vi "Get_Motor_Coordinates.vi"(6 "Microsteps (MS=64)":dbl=64.0, 9 "Output Unit":T1=enum."Micron", 11 "string":string) -> (0 "Motor 4 Coordinate (deg)":dbl, 1 "Motor 3 Coordinate":dbl, 2 "Motor 2 Coordinate":dbl, 3 "Motor 1 Coordinate":dbl)   [LabVIEW 2018]
uses:
  ConversionAndInformation/Unit_Control.ctl
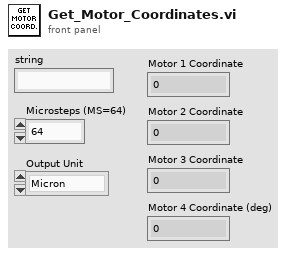
[diagram p1: front panel]
types:
  T1 = typedef "Unit_Control.ctl" = enum16{"Angle (Degrees)", "Rad", "Angle [TMC]", "Microsteps [TMC]", "Inches", "Nanometer", "Meter", "Centimeter", "Millimeter", "Micron"}
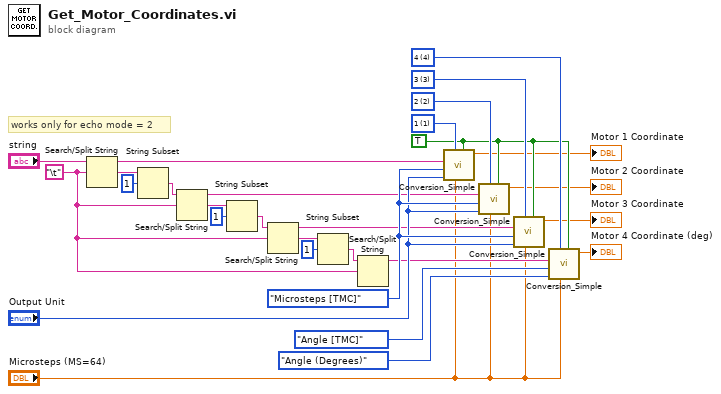
[diagram p0: block diagram]
diagram:
  w7 = u16 4 items=["none", "1", "2", "3", "4", "all"] ("Motor")
  w8 = u16 3 items=["none", "1", "2", "3", "4", "all"] ("Motor")
  w9 = u16 2 items=["none", "1", "2", "3", "4", "all"] ("Motor")
  w10 = u16 1 items=["none", "1", "2", "3", "4", "all"] ("Motor")
  w6 = TRUE ("Input = DBL/String (DBL[false])")
  w18 = Unit_Control."Microsteps [TMC]" ("Output Unit")
  w20 = "\t"
  # "works only for echo mode = 2"
  n1 = Search/Split String(string="string", search string/char (-)=w20) -> (substring before match=w14:string, match + rest of string=w29:string)  [unwired: 1 in, 1 out]
  n2 = String Subset(string=w29, offset (0)=1) -> (substring=w28:string)  [unwired: 1 in]
  n3 = Search/Split String(string=w28, search string/char (-)=w20) -> (substring before match=w13:string, match + rest of string=w26:string)  [unwired: 1 in, 1 out]
  n4 = String Subset(string=w26, offset (0)=1) -> (substring=w25:string)  [unwired: 1 in]
  n5 = Search/Split String(string=w25, search string/char (-)=w20) -> (substring before match=w12:string, match + rest of string=w22:string)  [unwired: 1 in, 1 out]
  n6 = String Subset(string=w22, offset (0)=1) -> (substring=w21:string)  [unwired: 1 in]
  n7 = Search/Split String(string=w21, search string/char (-)=w20) -> (substring before match=w11:string)  [unwired: 1 in, 2 out]
  n8 = call "Conversion_Simple.vi"("Input = DBL/String (DBL[false])"=w6, "Microsteps (MS=64)"="Microsteps (MS=64)", "Motor"=w10, "Output Unit"="Output Unit", "Input Unit"=w18, "Input String"=w14) -> ("Output"=→"Motor 1 Coordinate":dbl)  [unwired: 4 in, 1 out]
  n9 = call "Conversion_Simple.vi"("Input = DBL/String (DBL[false])"=w6, "Microsteps (MS=64)"="Microsteps (MS=64)", "Motor"=w9, "Output Unit"="Output Unit", "Input Unit"=w18, "Input String"=w13) -> ("Output"=→"Motor 2 Coordinate":dbl)  [unwired: 4 in, 1 out]
  n10 = call "Conversion_Simple.vi"("Input = DBL/String (DBL[false])"=w6, "Microsteps (MS=64)"="Microsteps (MS=64)", "Motor"=w8, "Output Unit"="Output Unit", "Input Unit"=w18, "Input String"=w12) -> ("Output"=→"Motor 3 Coordinate":dbl)  [unwired: 4 in, 1 out]
  n11 = call "Conversion_Simple.vi"("Input = DBL/String (DBL[false])"=w6, "Microsteps (MS=64)"="Microsteps (MS=64)", "Motor"=w7, "Output Unit"=Unit_Control."Angle (Degrees)", "Input Unit"=Unit_Control."Angle [TMC]" ("Output Unit"), "Input String"=w11) -> ("Output"=→"Motor 4 Coordinate (deg)":dbl)  [unwired: 4 in, 1 out]
